vi "Get all Object Item Offsets.vi"(8 "error in (no error)":errorcluster, 10 "Offset":i32, 11 "JSON":string) -> (0 "error out":errorcluster, 1 "Items":T1[](array[typedef]), 2 "Offset past Object":i32)   [LabVIEW 2019, in "JSONtext.lvlib"]
uses:
  JSONtext.lvlib
  Parsing/Found Items.ctl
  Parsing/Parsing State.ctl
  Parsing/Advance past Line Ending.vi
  Parsing/Advance past Number.vi
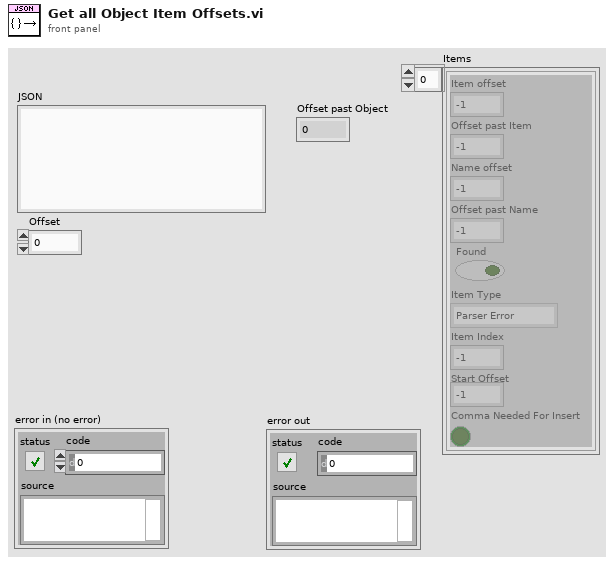
[diagram p1: front panel]
types:
  T1 = typedef "JSONtext.lvlib/Found Items.ctl" = cluster{"Item offset":i32, "Offset past Item":i32, "Name offset":i32, "Offset past Name":i32, "Found":bool, "Item Type":T2, "Item Index":i32, "Start Offset":i32, "Comma Needed For Insert":bool}
  T2 = typedef "JSONtext.lvlib/Parsing State.ctl" = enum16{"Parser Error", "Object", "Array", "String", "Number/Other", "Leading Whitespace", "Object end", "Array end", "Value end"}
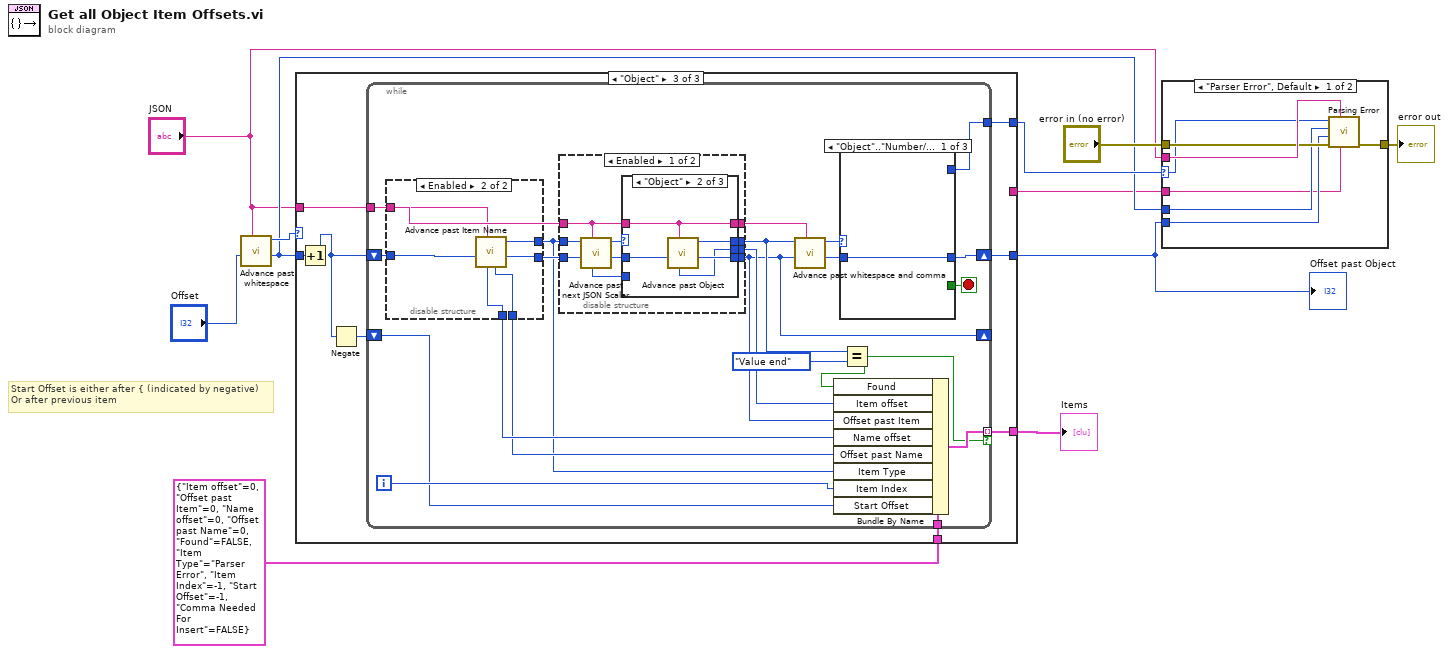
[diagram p0: block diagram]
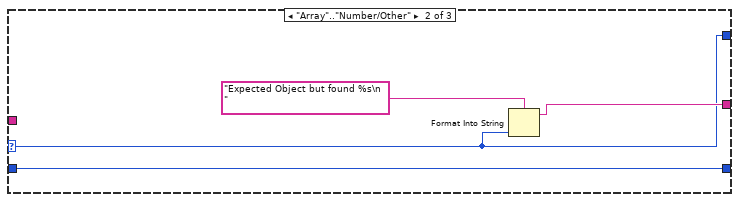
[diagram p3: hidden frame]
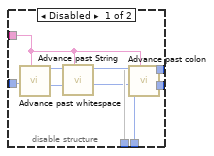
[diagram p4: hidden frame]
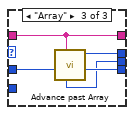
[diagram p6: hidden frame]
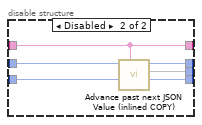
[diagram p7: hidden frame]
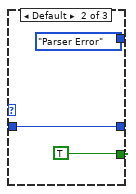
[diagram p8: hidden frame]
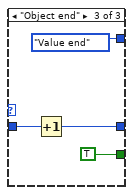
[diagram p9: hidden frame]
diagram:
  # "Start Offset is either after { (indicated by negative)\nOr after previous item"
  n1 = call "Advance past whitespace.vi"("JSON"="JSON", "Offset"="Offset") -> ("Offset of first non-whitespace"=w5:i32, "Parser State"=w10:T2)  [unwired: 7 in, 1 out]
  n2 = case shown="\"Object\"" w10 {
    selector: w10 -> [w13 w14 _]
    tunnel: [w13 w14 w25] -> w6
    tunnel: w5 -> [w12 w17 w24]
    tunnel: "JSON" -> [_ _ w23]
    tunnel: [w12 w17 w22] -> w7
    tunnel: [_ _ w21] -> w3
    tunnel: T1 {"Item offset"=0, "Offset past Item"=0, "Name offset"=0, "Offset past Name"=0, "Found"=FALSE, "Item Type"=enum."Parser Error", "Item Index"=-1, "Start Offset"=-1, "Comma Needed For Insert"=FALSE} -> [_ _ w20]
    tunnel: [_ w15 _] -> w1
    frame "Parser Error", Default {
    }
    frame "Array".."Number/Other" {
      n3 = Format Into String(format string="Expected Object but found %s\n " ("initial string"), w14) -> (resulting string=w15:string)  [unwired: 2 in, 1 out]
    }
    frame "Object" {
      n4 = Increment(x=w24) -> (x+1=w19:i32)
      n5 = Negate(x=w19) -> (-x=w18:i32)
      n6 = while {
        shift-right: [w44] -> w22
        shift-left: w19 -> [w41]
        tunnel: w23 -> [w38]
        tunnel: [w42] -> w25
        tunnel: [w34] -> w21 mode=indexing if=w33
        tunnel: w20 -> [w30]
        shift-right: [w27] -> _
        shift-left: w18 -> [w26]
        i -> [w28]
        stop <- w43 stop-if-true
        n7 = disable-structure shown="Enabled" {
          disable-tunnel: w41 -> [w54 w59]
          disable-tunnel: [w51 w61] -> w29
          disable-tunnel: [w50 w60] -> w39
          disable-tunnel: w38 -> [w49 w58]
          disable-tunnel: [w48 w57] -> w32
          disable-tunnel: [w47 w56] -> w31
          frame Disabled {
            n8 = call "Advance past whitespace.vi"("JSON"=w49, "Offset"=w54) -> ("Offset of first non-whitespace"=w53:i32, "Parser State"=w52:T2)  [unwired: 7 in, 1 out]
            n9 = call "Advance past String.vi"("JSON"=w49, "Offset"=w53, "State in"=w52) -> ("Offset past match"=w47:i32, 2:w48, "State"=w55:T2)  [unwired: 5 in, 1 out]
            n10 = call "Advance past colon.vi"("JSON"=w49, "Offset"=w47, "State"=w55) -> ("index"=w50:i32, "State"=w51:T2)  [unwired: 7 in]
          }
          frame Enabled {
            n11 = call "Advance past Item Name.vi"("JSON"=w58, "Offset"=w59) -> ("Offset past colon"=w60:i32, "State"=w61:T2, "Offset past Name"=w56:i32, "Name start out"=w57:i32)  [unwired: 6 in]
          }
        }
        n12 = disable-structure shown="Enabled" {
          disable-tunnel: [w71 w86] -> w40
          disable-tunnel: w29 -> [w69 w88]
          disable-tunnel: w39 -> [w68 w87]
          disable-tunnel: w38 -> [w66 w86]
          disable-tunnel: [w65 w89] -> w37
          disable-tunnel: [w64 w90] -> w35
          disable-tunnel: [w63 w91] -> w27
          frame Enabled {
            n13 = call "Advance past next JSON Scaler.vi"("JSON"=w66, "Offset"=w68, "Parser State in"=w69) -> ("Offset Past"=w67:i32, "Parser State"=w70:T2, "Value start"=w62:i32)  [unwired: 6 in]
            n14 = case shown="\"Object\"" w70 {
              selector: w70 -> [w74 _ _]
              tunnel: w67 -> [w73 w80 w85]
              tunnel: [w74 w79 w84] -> w65
              tunnel: [w73 w78 w83] -> w63
              tunnel: w66 -> [w75 w77 w82]
              tunnel: [w75 w77 w82] -> w71
              tunnel: [w72 w76 w81] -> w64
              tunnel: w62 -> [w72 _ _]
              frame Default {
              }
              frame "Object" {
                n15 = call "Advance past Object.vi"("JSON"=w77, "Offset"=w80) -> ("Offset past Object"=w78:i32, "State"=w79:T2, "Object Start"=w76:i32)  [unwired: 7 in]
              }
              frame "Array" {
                n16 = call "Advance past Array.vi"("JSON"=w82, "Offset"=w85) -> ("Offset past Array"=w83:i32, "State"=w84:T2, "Array Start"=w81:i32)  [unwired: 6 in, 1 out]
              }
            }
          }
          frame Disabled {
            n17 = call "Advance past next JSON Value (inlined COPY).vi"("JSON"=w86, "Offset"=w87, "State"=w88) -> ("Offset"=w91:i32, 2:w90, "State"=w89:T2)  [unwired: 3 in, 3 out]
          }
        }
        n18 = call "Advance past whitespace and comma.vi"("JSON"=w40, "Offset"=w27, "State in"=w37) -> ("Offset past match"=w46:i32, "State"=w45:T2)  [unwired: 6 in, 1 out]
        n19 = case shown="\"Object\"..\"Number/Other\"" w45 {
          tunnel: [_ TRUE TRUE] -> w43
          tunnel: [_ Parsing_State."Parser Error" Parsing_State."Value end"] -> w42
          tunnel: w46 -> [w92 w93 w97]
          tunnel: [w92 w93 w96] -> w44
          frame "Object".."Number/Other" {
          }
          frame Default {
          }
          frame "Object end" {
            n20 = Increment(x=w97) -> (x+1=w96:i32)
          }
        }
        n21 = Equal?(x=w37, y=Parsing_State."Value end") -> (x = y?=w33:bool)
        n22 = Bundle By Name(cluster=w30, "Found"=w33, "Item offset"=w35, "Offset past Item"=w27, "Name offset"=w32, "Offset past Name"=w31, "Item Type"=w29, "Item Index"=w28, "Start Offset"=w26) -> (w34:T1)
      }
    }
  }
  "Offset past Object" <- w7
  "Items" <- w3
  n23 = case shown="\"Parser Error\", Default" w6 {
    selector: w6 -> [w101 _]
    tunnel: "JSON" -> [w106 _]
    tunnel: "error in (no error)" -> [w105 w107]
    tunnel: [w104 w107] -> w9
    tunnel: w5 -> [w103 _]
    tunnel: w7 -> [w102 _]
    tunnel: w1 -> [w100 _]
    frame "Parser Error", Default {
      n24 = call "Parsing Error.vi"("initial string"=w100, "JSON"=w106, "error in (no error)"=w105, "Offset past match"=w102, "Value start"=w103, "State"=w101) -> ("error out"=w104:errorcluster)  [unwired: 5 in]
    }
    frame "Value end" {
    }
  }
  "error out" <- w9
